vi "Programme.vi"() -> ()   [LabVIEW 2015]
uses:
  <vilib>/Analysis/2dsp.llb/Real FFT.vi
  <vilib>/express/express analysis/Spectral/Block/exnSpectralBlock spectral measurements peak poly.vi
  <vilib>/express/express analysis/Spectral/Block/exnSpectralBlock spectral measurements peak DDT.vi
  <vilib>/express/express analysis/Spectral/XNode/ExpressSpectralMeasurementsBlockNode.xnode
  <vilib>/Analysis/NI_AALPro.lvlib
panel:
  out "Mixed Signal Graph":dbl[][](graph)
  in  "FFT size":i32
  in  "stop":bool
  in  "stop (T)":bool=TRUE
  in  "timeout (s)":dbl=10.0 format="%0.2f"
  in  "number of samples":i32=100
  in  "rate":dbl=1000.0
  out "data":dynamicdata(graph)
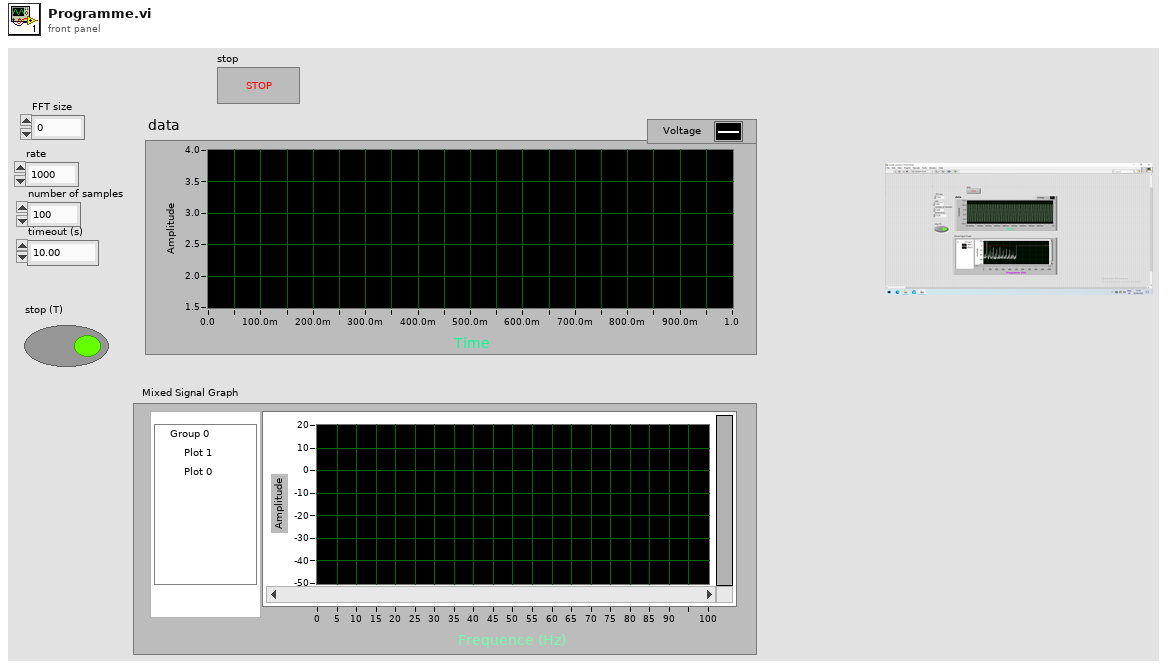
[diagram p1: front panel]
types:
  T1 = cluster{"averaging mode":u16, "weighting mode":u16, "number of averages":u32}
  T2 = cluster{"dB On (F)":bool, "unwrap phase (F)":bool, "convert to degree (F)":bool}
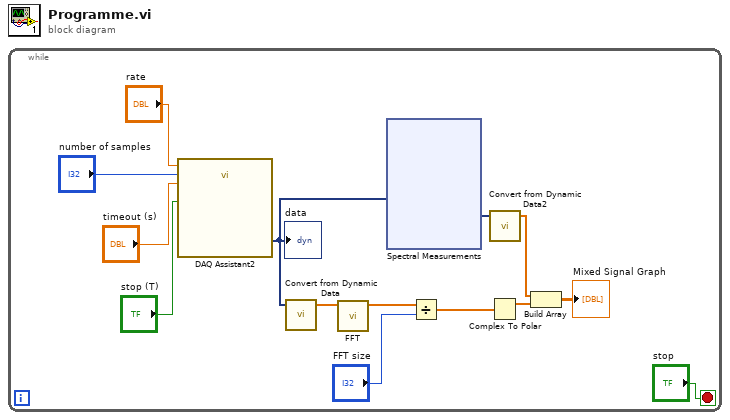
[diagram p0: block diagram]
diagram:
  n1 = while {
    stop <- "stop" stop-if-true
    n2 = call "DAQ Assistant2"("rate"="rate", "number of samples"="number of samples", "timeout (s)"="timeout (s)", "stop (T)"="stop (T)") -> ("data"=w5:dynamicdata)  [unwired: 13 in, 2 out]
    "data" <- w5
    n3 = call "Convert from Dynamic Data"("Dynamic Data Type"=w5) -> ("Array"=w13:dbl[])  [unwired: 3 in]
    n4 = call-poly <vilib>:"FFT.vi"("X"=w13) -> ("FFT {X}"=w12:cdb[])  [unwired: 9 in, 1 out]
    n5 = xnode "Spectral Measurements"("Signals"=w5) -> ("FFT - (Peak)"=w8:dynamicdata)  [unwired: 1 in, 2 out]
    n6 = Divide(x=w12, y="FFT size") -> (x/y=w10:cdb[])
    n7 = call "Convert from Dynamic Data2"("Dynamic Data Type"=w8) -> ("Array"=w7:dbl[])  [unwired: 3 in]
    n8 = Complex To Polar(r * e^(i*theta)=w10) -> (r=w9:dbl[])  [unwired: 1 out]
    n9 = Build Array(w7, w9) -> (→"Mixed Signal Graph":dbl[][])
  }
